vi "start_data_file.vi"(0 "sample id":string, 1 "volume (mL)":dbl, 2 "DataFile":path, 3 "File Header Settings":T2={"Flow Rate"="", "Operator"="", "Sample Type"="Unknown"}, 4 "iteration":dbl) -> (5 "file session out":T1)   [LabVIEW 2010]
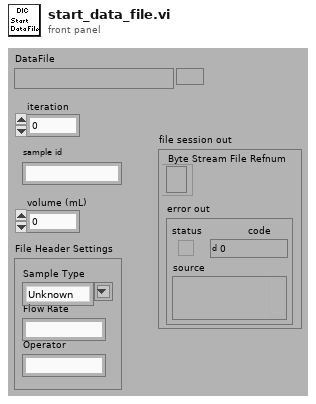
[diagram p1: front panel]
types:
  T1 = cluster{"Byte Stream File Refnum":refnum<file>, "error out":errorcluster}
  T2 = cluster{"Flow Rate":string, "Operator":string, "Sample Type":string}
  T3 = cluster{"refnum out":refnum<file>, "error out":errorcluster}
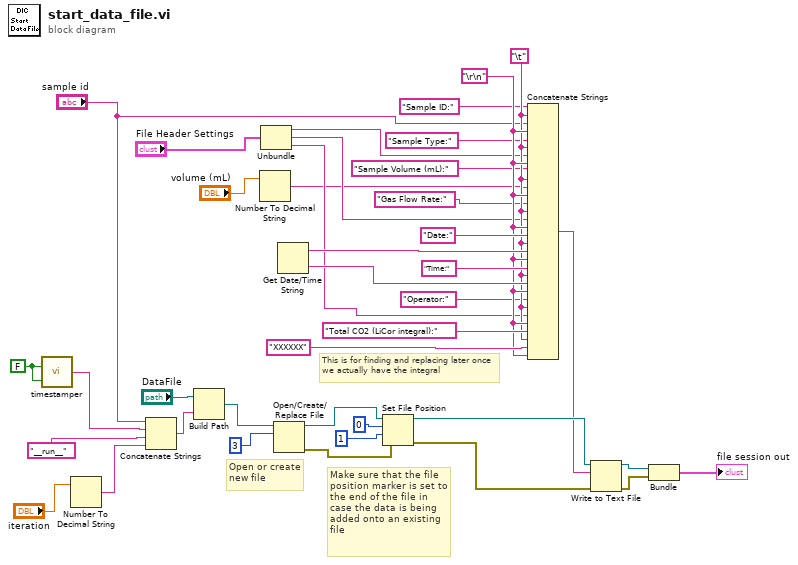
[diagram p0: block diagram]
diagram:
  w19 = FALSE
  w15 = "\t"
  w16 = "\r\n"
  # "This is for finding and replacing later once we actually have the integral"
  # "Make sure that the file position marker is set to the end of the file in case the data is being added onto an existing file"
  # "Open or create new file"
  n1 = call "timestamper.vi"("seconds?"=w19, "ms?"=w19) -> ("datetime output"=w18:string)
  n2 = Number To Decimal String(number="iteration") -> (decimal integer string=w37:string)  [unwired: 1 in]
  n3 = Concatenate Strings("sample id", w18, "__run__", w37) -> (w36:string)
  n4 = Build Path(base path="DataFile", name or relative path=w36) -> (appended path=w35:path)
  n5 = Number To Decimal String(number="volume (mL)") -> (decimal integer string=w1:string)  [unwired: 1 in]
  n6 = Unbundle("File Header Settings") -> ("Flow Rate"=w4:string, "Operator"=w3:string, "Sample Type"=w9:string)
  n7 = Open/Create/Replace File(file path (use dialog)=w35, operation (0:open)=3) -> (refnum out=w28:refnum<file>, error out=w31:errorcluster)  [unwired: 4 in, 1 out]
  n8 = Get Date/Time String() -> (date string=w26:string, time string=w24:string)  [unwired: 3 in]
  n9 = Set File Position(offset (in bytes) (0)=0, refnum=w28, from (0:start)=1, error in=w31) -> (refnum out=w29:refnum<file>, error out=w30:errorcluster)
  n10 = Concatenate Strings("Sample ID:", w15, "sample id", w16, "Sample Type:", w15, w4, w16, "Sample Volume (mL):", w15, w1, w16, "Gas Flow Rate:", w15, w3, w16, "Date:", w15, w26, w16, "Time:", w15, w24, w16, "Operator:", w15, w9, w16, "Total CO2 (LiCor integral):", w15, "XXXXXX", w16) -> (w22:string)
  n11 = Write to Text File(file (use dialog)=w29, text=w22, error in=w30) -> (refnum out=w7:refnum<file>, error out=w6:errorcluster)  [unwired: 1 in, 1 out]
  n12 = Bundle("refnum out"=w7, "error out"=w6) -> (→"file session out":T3)  [unwired: 1 in]
